vi "Get AER vectors.vi"(10 "ID [i]":i32, 11 "AER in":refnum<class "AER.lvclass">) -> (0 "PreIDs [i]":i32[](array[numeric]), 1 "Acc NoPre [i-1]":i32, 2 "NoPre [i-1]":i32[](array[numeric]), 3 "AER out":refnum<class "AER.lvclass">, 4 "W[i]":dbl[](array[numeric]), 5 "NoPre [i]":i32)   [LabVIEW 2016, in "AER.lvclass"]
doc: "This Vi reads the NoPre, the PreIds of the input neuron from the AER table"
uses:
  AER.lvclass
  AER.lvclass/AER.ctl
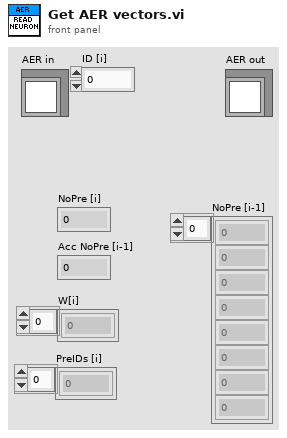
[diagram p1: front panel]
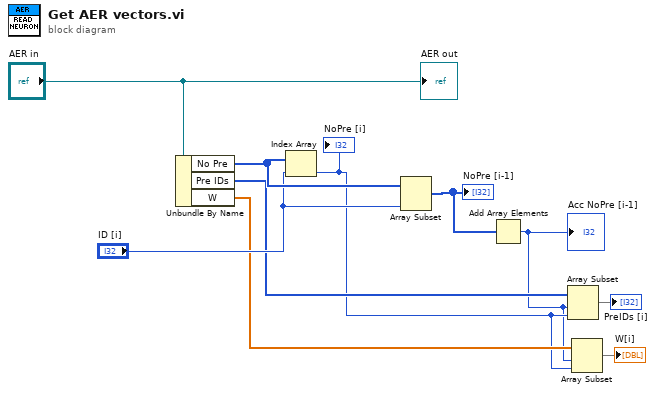
[diagram p0: block diagram]
diagram:
  n1 = Unbundle By Name("AER in") -> ("No Pre"=w9:i32[], "Pre IDs"=w6:i32[], "W"=w4:dbl[])
  n2 = Index Array(array=w9, index="ID [i]") -> (element=w3:i32)
  "NoPre [i]" <- w3
  n3 = Array Subset(array=w9, length="ID [i]") -> (w8:i32[])  [unwired: 1 in]
  "NoPre [i-1]" <- w8
  n4 = Add Array Elements(numeric array=w8) -> (sum=w1:i32)
  "Acc NoPre [i-1]" <- w1
  n5 = Array Subset(array=w6, index=w1, length=w3) -> (→"PreIDs [i]":i32[])
  n6 = Array Subset(array=w4, index=w1, length=w3) -> (→"W[i]":dbl[])
  "AER out" <- "AER in"
